vi "Get Keywords.vi"(8 "error in (no error)":errorcluster, 11 "String Functions in":refnum<class "String Functions.lvclass">) -> (0 "error out":errorcluster, 2 "Keywords":string[](array[string]), 3 "String Functions out":refnum<class "String Functions.lvclass">)   [LabVIEW 2019, in "String Functions.lvclass"]
uses:
  String Functions.lvclass
  functionsbase/functionbase.lvclass
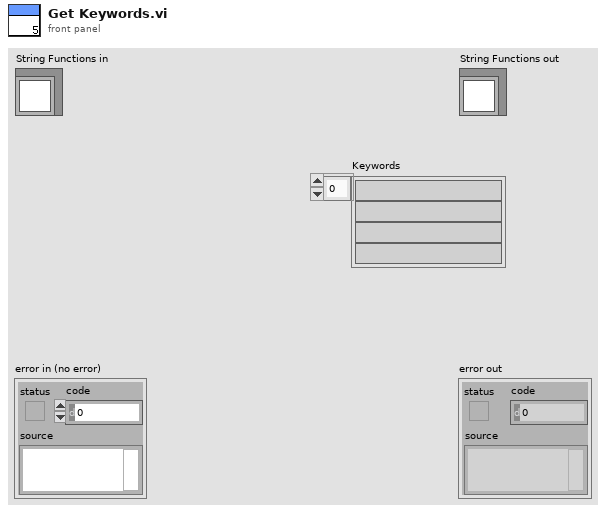
[diagram p1: front panel]
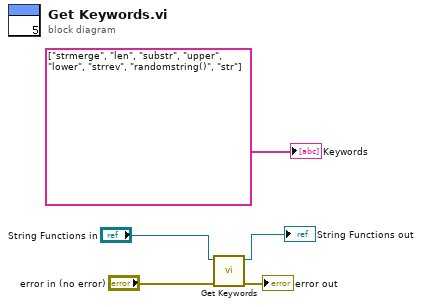
[diagram p0: block diagram]
diagram:
  n1 = call-parent "Get Keywords.vi"("error in (no error)"="error in (no error)", "functionbase in"="String Functions in") -> ("error out"=→"error out":errorcluster, "functionbase out"=→"String Functions out":refnum<class "String Functions.lvclass">)  [unwired: 7 in, 1 out]
  "Keywords" <- string[] ["strmerge", "len", "substr", "upper", "lower", "strrev", "randomstring()", "str"] ("Keywords")
